vi "Kal Daten kopieren.vi"(11 "Komponente":i32) -> (1 "Ziel MB":i32[](array[numeric]), 3 "Kalibrierter MB":i32)   [LabVIEW 2020, in "Auto Kalibrieren.lvlib"]
uses:
  Auto Kalibrieren.lvlib
  Analysator Definition/FGV Analysator Definition Aktionen.ctl
  Analysator Definition/Analysator Definition.lvlib
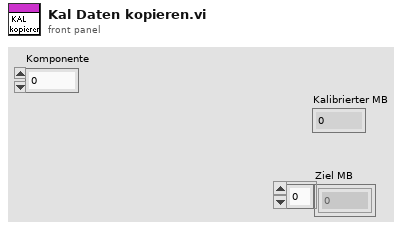
[diagram p1: front panel]
types:
  T1 = typedef "Analysator Definition.lvlib/FGV Analysator Definition Aktionen.ctl" = enum16{"lesen", "MB setzen", "MB KAL setzen", "laden"}
  T2 = typedef "Analysator Definition.lvlib/Betriebsdaten Komponente.ctl" = cluster{"Namen":string[], "MB Namen":string[], "Einheit":string, "MB Aktuell":u16, "MB Endwert":u16, "CalGase":u16[], "MB für KAL":u16[], "CG für KAL":u16[]}
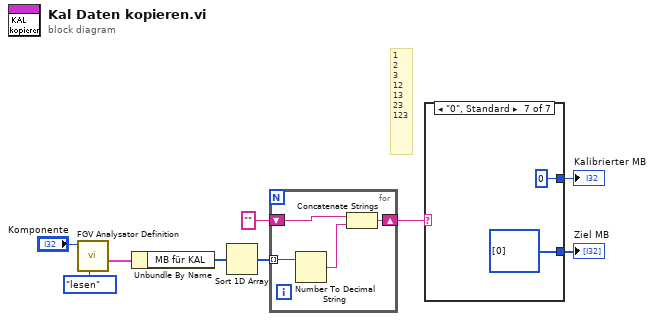
[diagram p0: block diagram]
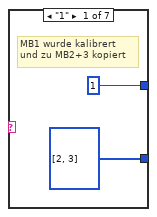
[diagram p2: hidden frame]
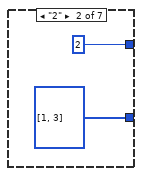
[diagram p3: hidden frame]
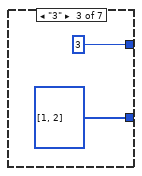
[diagram p4: hidden frame]
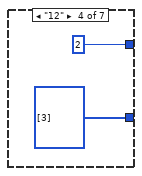
[diagram p5: hidden frame]
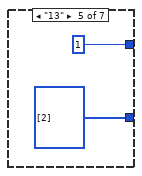
[diagram p6: hidden frame]
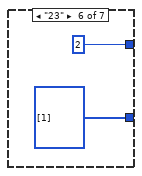
[diagram p7: hidden frame]
diagram:
  # "1 \n2\n3\n12\n13\n23\n123"
  n1 = call "FGV Analysator Definition.vi"("Aktionen"=FGV_Analysator_Definition_Aktionen."lesen", "Komponente"="Komponente") -> ("Betriebsdaten Komponente"=w2:T2)  [unwired: 5 in, 4 out]
  n2 = Unbundle By Name(w2) -> ("MB für KAL"=w8:u16[])
  n3 = Sort 1D Array(array=w8) -> (sorted array=w7:u16[])
  n4 = for {
    tunnel: w7 -> [w13] mode=indexing
    shift-right: [w11] -> w6
    shift-left: "" -> [w12]
    n5 = Number To Decimal String(number=w13) -> (decimal integer string=w10:string)  [unwired: 1 in]
    n6 = Concatenate Strings(w12, w10) -> (w11:string)
  }
  n7 = case shown="\"0\", Standard" w6 {
    tunnel: [i32[] [2, 3] i32[] [1, 3] i32[] [1, 2] i32[] [3] i32[] [2] i32[] [1] i32[] [0]] -> w4
    tunnel: [1 ("Index") 2 ("Index") 3 ("Index") 2 ("Index") 1 ("Index") 2 ("Index") 0 ("Index")] -> w5
    frame "1" {
      # "MB1 wurde kalibrert\nund zu MB2+3 kopiert"
    }
    frame "2" {
    }
    frame "3" {
    }
    frame "12" {
    }
    frame "13" {
    }
    frame "23" {
    }
    frame "0", Default {
    }
  }
  "Kalibrierter MB" <- w5
  "Ziel MB" <- w4
